vi "SG90_Servo.vi"(10 "Frequency (Hz)":dbl, 11 "Position":dbl) -> (1 "Duty Cycle (to drive RIO PWM)":dbl, 2 "Duty Cycle %":dbl, 3 "Pulse Width (ms)":dbl)   [LabVIEW 2021]
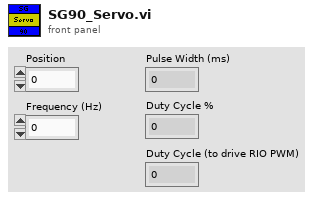
[diagram p1: front panel]
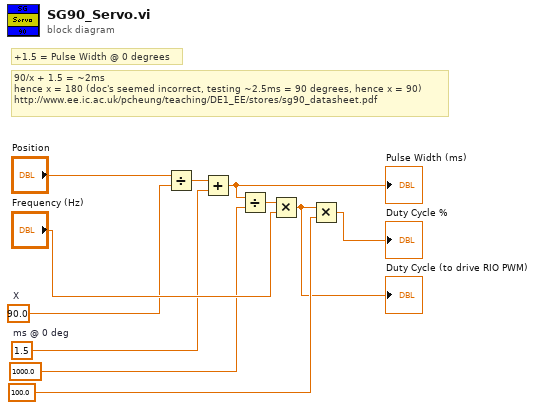
[diagram p0: block diagram]
diagram:
  w4 = 1.5  # ms @ 0 deg
  w2 = 90.0  # X
  # "+1.5 = Pulse Width @ 0 degrees"
  # "90/x + 1.5 = ~2ms\nhence x = 180 (doc's seemed incorrect, testing ~2.5ms = 90 degrees, hence x = 90)\nhttp://www.ee.ic.ac.uk/pcheung/teaching/DE1_EE/stores/sg90_datasheet.pdf"
  n1 = Divide(x="Position", y=w2) -> (x/y=w3:dbl)
  n2 = Add(x=w3, y=w4) -> (x+y=w5:dbl)
  "Pulse Width (ms)" <- w5
  n3 = Divide(x=w5, y=1000.0) -> (x/y=w7:dbl)
  n4 = Multiply(x=w7, y="Frequency (Hz)") -> (x*y=w9:dbl)
  "Duty Cycle (to drive RIO PWM)" <- w9
  n5 = Multiply(x=w9, y=100.0) -> (x*y=→"Duty Cycle %":dbl)
